vi "New LabVIEW File.vi"(8 "error in (no error)":errorcluster, 10 "Path":path) -> (0 "error out":errorcluster, 3 "LabVIEW File out":refnum<class "LabVIEW File.lvclass">)   [LabVIEW 2020, in "Save for Previous Version.lvlib" / "LabVIEW File.lvclass"]
uses:
  LabVIEW File.lvclass
  \\Mac\Home/JKI/GitHub/save-for-previous-labview-version/source/File/File.lvclass/File.lvclass
  VI File/VI File.lvclass
  \\Mac\Home/JKI/GitHub/save-for-previous-labview-version/source/LabVIEW File/LabVIEW File.lvclass
  LabVIEW Project File/LabVIEW Project File.lvclass
  LabVIEW File.lvclass/LabVIEW File.ctl
  File/File.lvclass/File.lvclass/File.ctl
  Write Version String.vi
  Write Version Number.vi
  File/File.lvclass/Write Path.vi
  Write LabVIEW File Type.vi
  <vilib>/Utility/lvfile.llb/NI_FileType.lvlib
  LabVIEW Library File/LabVIEW Library File.lvclass
  \\Mac\Home/JKI/GitHub/save-for-previous-labview-version/source/VI File/VI File.lvclass
  \\Mac\Home/JKI/GitHub/save-for-previous-labview-version/source/LabVIEW Project File/LabVIEW Project File.lvclass
  \\Mac\Home/JKI/GitHub/save-for-previous-labview-version/source/LabVIEW Library File/LabVIEW Library File.lvclass
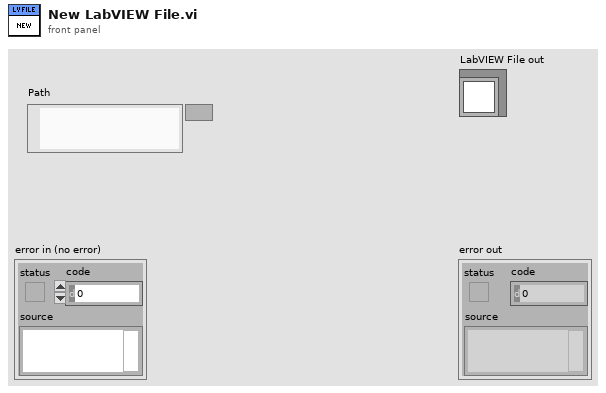
[diagram p1: front panel]
types:
  T1 = typedef "NI_FileType.lvlib/FT_FileTypes.ctl" = enum32{"Invalid file/path", "Unknown type", "Instrument", "Control", "Polymorphic VI", "Project", "Library", "LVClass", "XControl", "XNode", "CIN", "Run-time menu", "Palette menu", "LLB", "Shortcut", "Directory", "Class Private Data Control", "Statechart", "MathScript .m file", "Ladder Diagram", "LVLibp"}
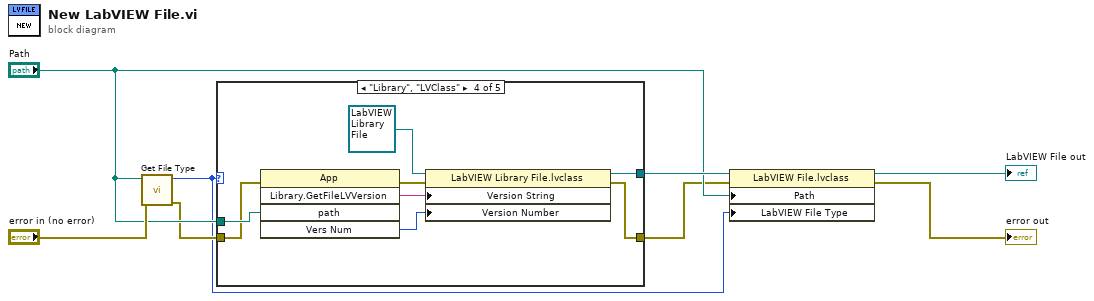
[diagram p0: block diagram]
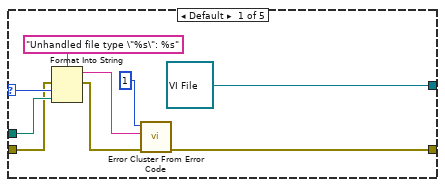
[diagram p2: hidden frame]
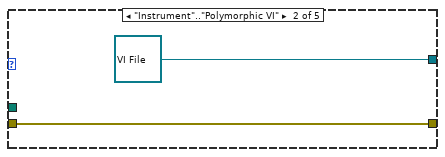
[diagram p3: hidden frame]
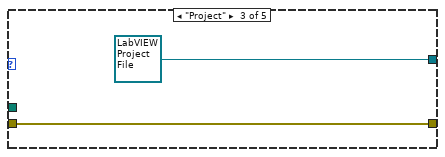
[diagram p4: hidden frame]
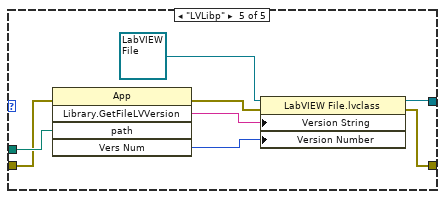
[diagram p5: hidden frame]
diagram:
  n1 = call <vilib>:"Get File Type.vi"("error in (no error)"="error in (no error)", "path"="Path") -> ("error out"=w2:errorcluster, "file type"=w1:T1)  [unwired: 7 in, 1 out]
  n2 = case shown="\"Library\", \"LVClass\"" w1 {
    selector: w1 -> [w14 _ _ _ _]
    tunnel: [refnum<class "VI File.lvclass"> refnum ("Save for Previous Version.lvlib:VI File.lvclass") refnum<class "VI File.lvclass"> refnum ("Save for Previous Version.lvlib:VI File.lvclass") refnum<class "LabVIEW Project File.lvclass"> refnum ("Save for Previous Version.lvlib:LabVIEW Project File.lvclass") w28 w36] -> w7
    tunnel: [w16 w18 w20 w23 w31] -> w4
    tunnel: w2 -> [w9 w18 w20 w24 w32]
    tunnel: "Path" -> [w13 _ _ w29 w37]
    frame Default {
      n3 = Format Into String(format string="Unhandled file type \"%s\": %s", error in=w9, w14, w13) -> (resulting string=w11:string, error out=w10:errorcluster)  [unwired: 1 in]
      n4 = call <vilib>:"Error Cluster From Error Code.vi"("error in (no error)"=w10, "error message (\"\")"=w11, "error code (0)"=1) -> ("error out"=w16:errorcluster)  [unwired: 6 in]
    }
    frame "Instrument".."Polymorphic VI" {
    }
    frame "Project" {
    }
    frame "Library", "LVClass" {
      n5 = invoke class="App" method="Library.GetFileLVVersion"(error in=w24, "path"=w29) -> (error out=w25:errorcluster, "Library.GetFileLVVersion"=w26:string, "Vers Num"=w27:u32)  [unwired: 3 in, 2 out]
      n6 = property class="LabVIEW Library File.lvclass"(reference=refnum<class "LabVIEW Library File.lvclass"> refnum, error in=w25, "Version String"=w26, "Version Number"=w27) -> (reference out=w28:refnum<class "LabVIEW Library File.lvclass">, error out=w23:errorcluster)
    }
    frame "LVLibp" {
      n7 = invoke class="App" method="Library.GetFileLVVersion"(error in=w32, "path"=w37) -> (error out=w33:errorcluster, "Library.GetFileLVVersion"=w34:string, "Vers Num"=w35:u32)  [unwired: 3 in, 2 out]
      n8 = property class="LabVIEW File.lvclass"(reference=refnum<class "LabVIEW File.lvclass"> refnum, error in=w33, "Version String"=w34, "Version Number"=w35) -> (reference out=w36:refnum<class "LabVIEW File.lvclass">, error out=w31:errorcluster)
    }
  }
  n9 = property class="LabVIEW File.lvclass"(reference=w7, error in=w4, "Path"="Path", "LabVIEW File Type"=w1) -> (reference out=→"LabVIEW File out":refnum<class "LabVIEW File.lvclass">, error out=→"error out":errorcluster)
